vi "estimateKalmanRP.vi"(0 "Vision in":refnum<class "Vision.lvclass">, 1 "Robot ID":u32, 3 "Camera_id":enum16{"3", "2", "1", "0"}(ring), 4 "Click To continue":bool, 6 "Field Size":T2, 7 "Number of\nmeasurements\nper point":i32=1000, 9 "Team":enum16{"Azul", "Amarelo"}(ring) caption="Enum", 10 "NewCameras":T5[](array[typedef]) {"robots_blue"."height" format="%+4.3f"; "robots_blue"."pixel_y" format="%+4.3f"; "robots_blue"."pixel_x" format="%+4.3f"; "robots_blue"."orientation" format="%+4.3f"; "robots_blue"."y" format="%+4.3f"; "robots_blue"."confidence" format="%4.3f"; "robots_blue"."x" format="%+4.3f"; "robots_yellow"."height" format="%+4.3f"; "robots_yellow"."pixel_y" format="%+4.3f"; "robots_yellow"."pixel_x" format="%+4.3f"; "robots_yellow"."orientation" format="%+4.3f"; "robots_yellow"."y" format="%+4.3f"; "robots_yellow"."confidence" format="%4.3f"; "robots_yellow"."x" format="%+4.3f"}, 16 "ID Cameras Array":dbl[](array[numeric])) -> (11 "Current State":T3=enum."Canto inferior direito", 13 "Next State":T3=enum."Canto inferior direito", 14 "Vision out":refnum<class "Vision.lvclass">, 15 "Point Finished?":bool, 17 "Camera Finished?":bool, 18 "covariance matrix R":T4, 19 "covariance matrix P":T4)   [LabVIEW 2018, in "Vision.lvclass"]
uses:
  Vision.lvclass
  Old vision/Controls/SSL Detection Frame.ctl
  Old vision/Controls/SSL Detection Robot.ctl
  <vilib>/Analysis/Matrix/Datatypes/RealMatrix.ctl
  Old vision/Controls/SSL Detection Ball.ctl
  EstimateState.ctl
  EstimateLocation.ctl
  <vilib>/gmath/NI_Gmath.lvlib
  <vilib>/Analysis/Matrix/NI_Matrix.lvlib
panel:
  in  "Local":T1
  out "error out":errorcluster
  in  "error in (no error)":errorcluster
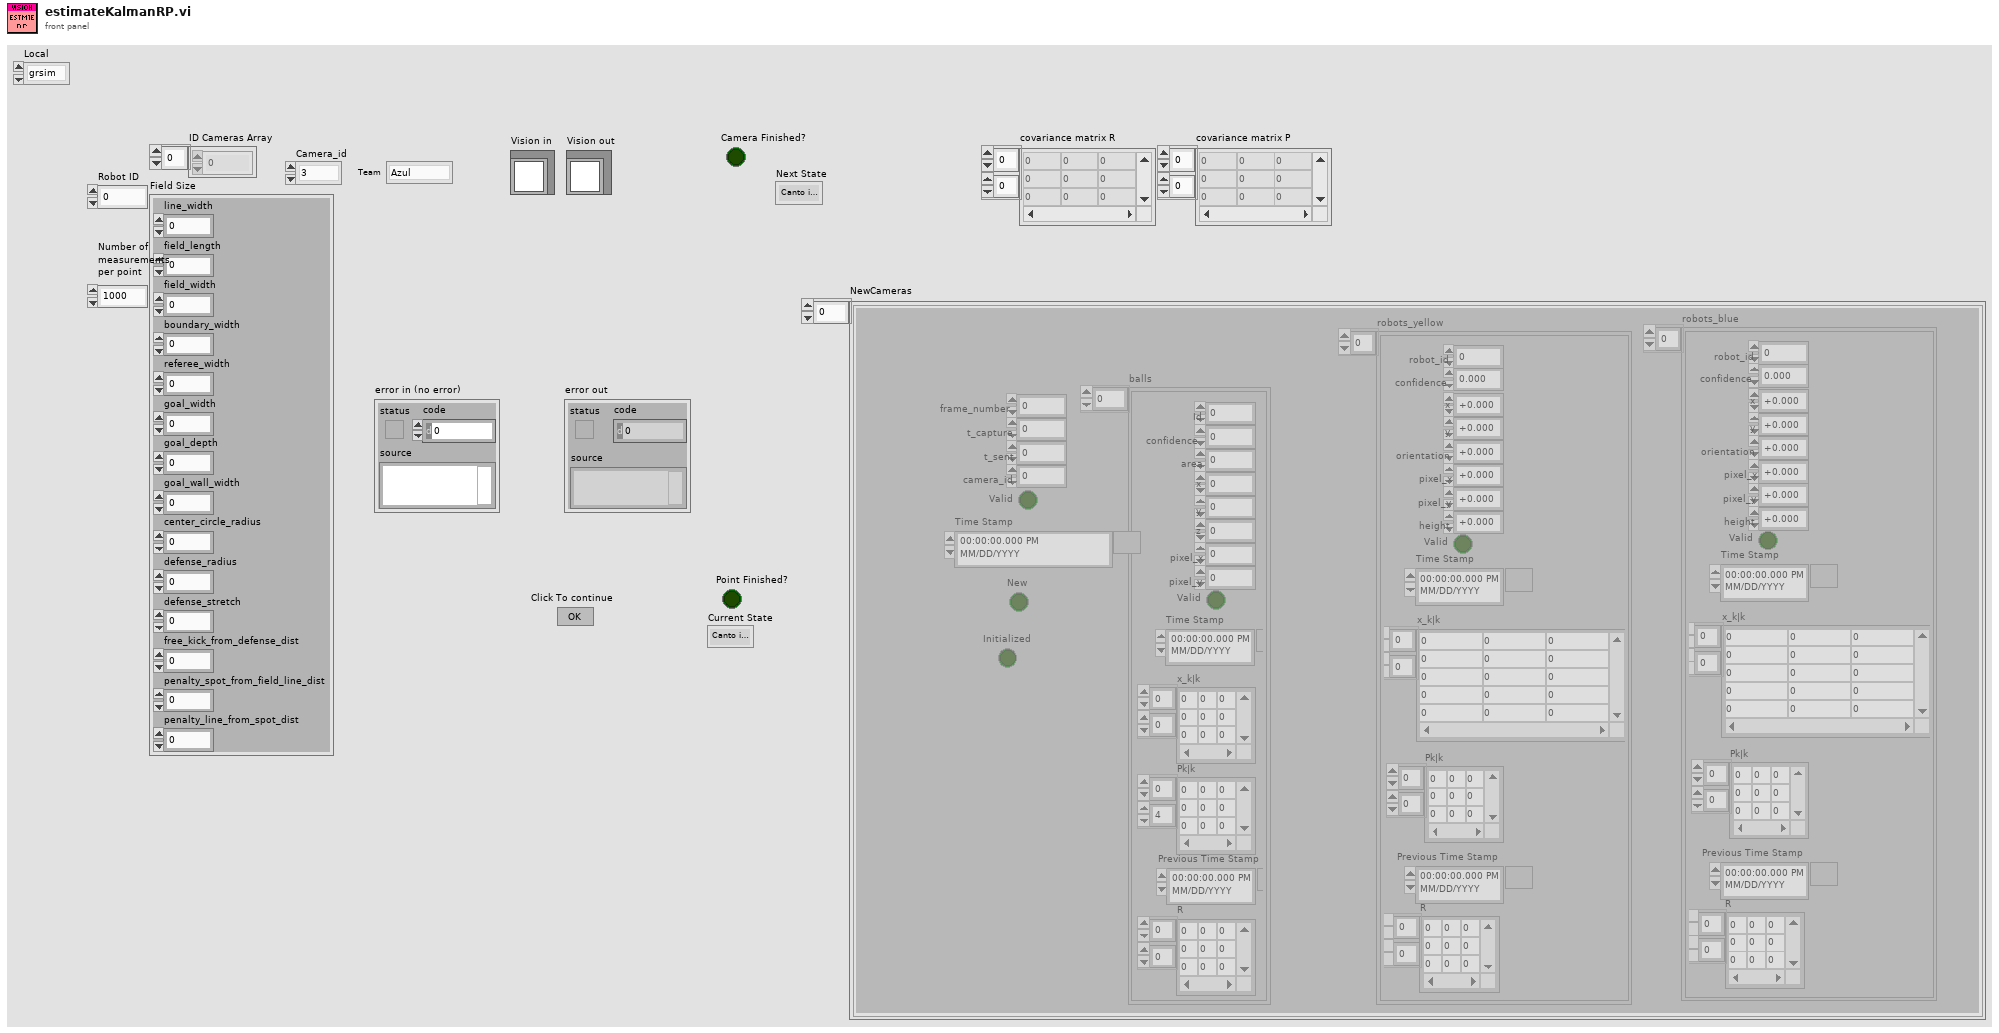
[diagram p1: front panel]
types:
  T1 = typedef "EstimateLocation.ctl" = enum16{"grsim", "RoboCup", "LARC"}
  T2 = cluster{"line_width":u32, "field_length":u32, "field_width":u32, "boundary_width":u32, "referee_width":u32, "goal_width":u32, "goal_depth":u32, "goal_wall_width":u32, "center_circle_radius":u32, "defense_radius":u32, "defense_stretch":u32, "free_kick_from_defense_dist":u32, "penalty_spot_from_field_line_dist":u32, "penalty_line_from_spot_dist":u32}
  T3 = typedef "EstimateState.ctl" = enum16{"Terminado", "Calculando", "Aguardando início", "Aguardando próximo passo", "Canto inferior direito", "Centro do gol direito", "Canto superior direito", "Meio superior", "Canto superior esquerdo", "Meio inferior", "Meio do campo", "Centro do gol esquerdo", "Canto inferior esquerdo", "Abaixo da câmera"}
  T4 = typedef "NI_Matrix.lvlib/RealMatrix.ctl" = dbl[][]
  T5 = typedef "SSL Detection Frame.ctl" = cluster{"frame_number":u32, "t_capture":dbl, "t_sent":dbl, "camera_id":u32, "robots_yellow":T6[], "robots_blue":T6[], "balls":T7[], "Valid":bool, "Time Stamp":timestamp, "New":bool, "Initialized":bool}
  T6 = typedef "SSL Detection Robot.ctl" = cluster{"x":sgl, "robot_id":u32, "confidence":sgl, "y":sgl, "orientation":sgl, "pixel_x":sgl, "pixel_y":sgl, "height":sgl, "Valid":bool, "Time Stamp":timestamp, "x_k|k":T4, "Pk|k":T4, "Previous Time Stamp":timestamp, "R":T4}
  T7 = typedef "SSL Detection Ball.ctl" = cluster{"x":sgl, "area":u32, "confidence":sgl, "y":sgl, "z":sgl, "pixel_x":sgl, "pixel_y":sgl, "Valid":bool, "Time Stamp":timestamp, "x_k|k":T4, "Pk|k":T4, "Id":u32, "Previous Time Stamp":timestamp, "R":T4}
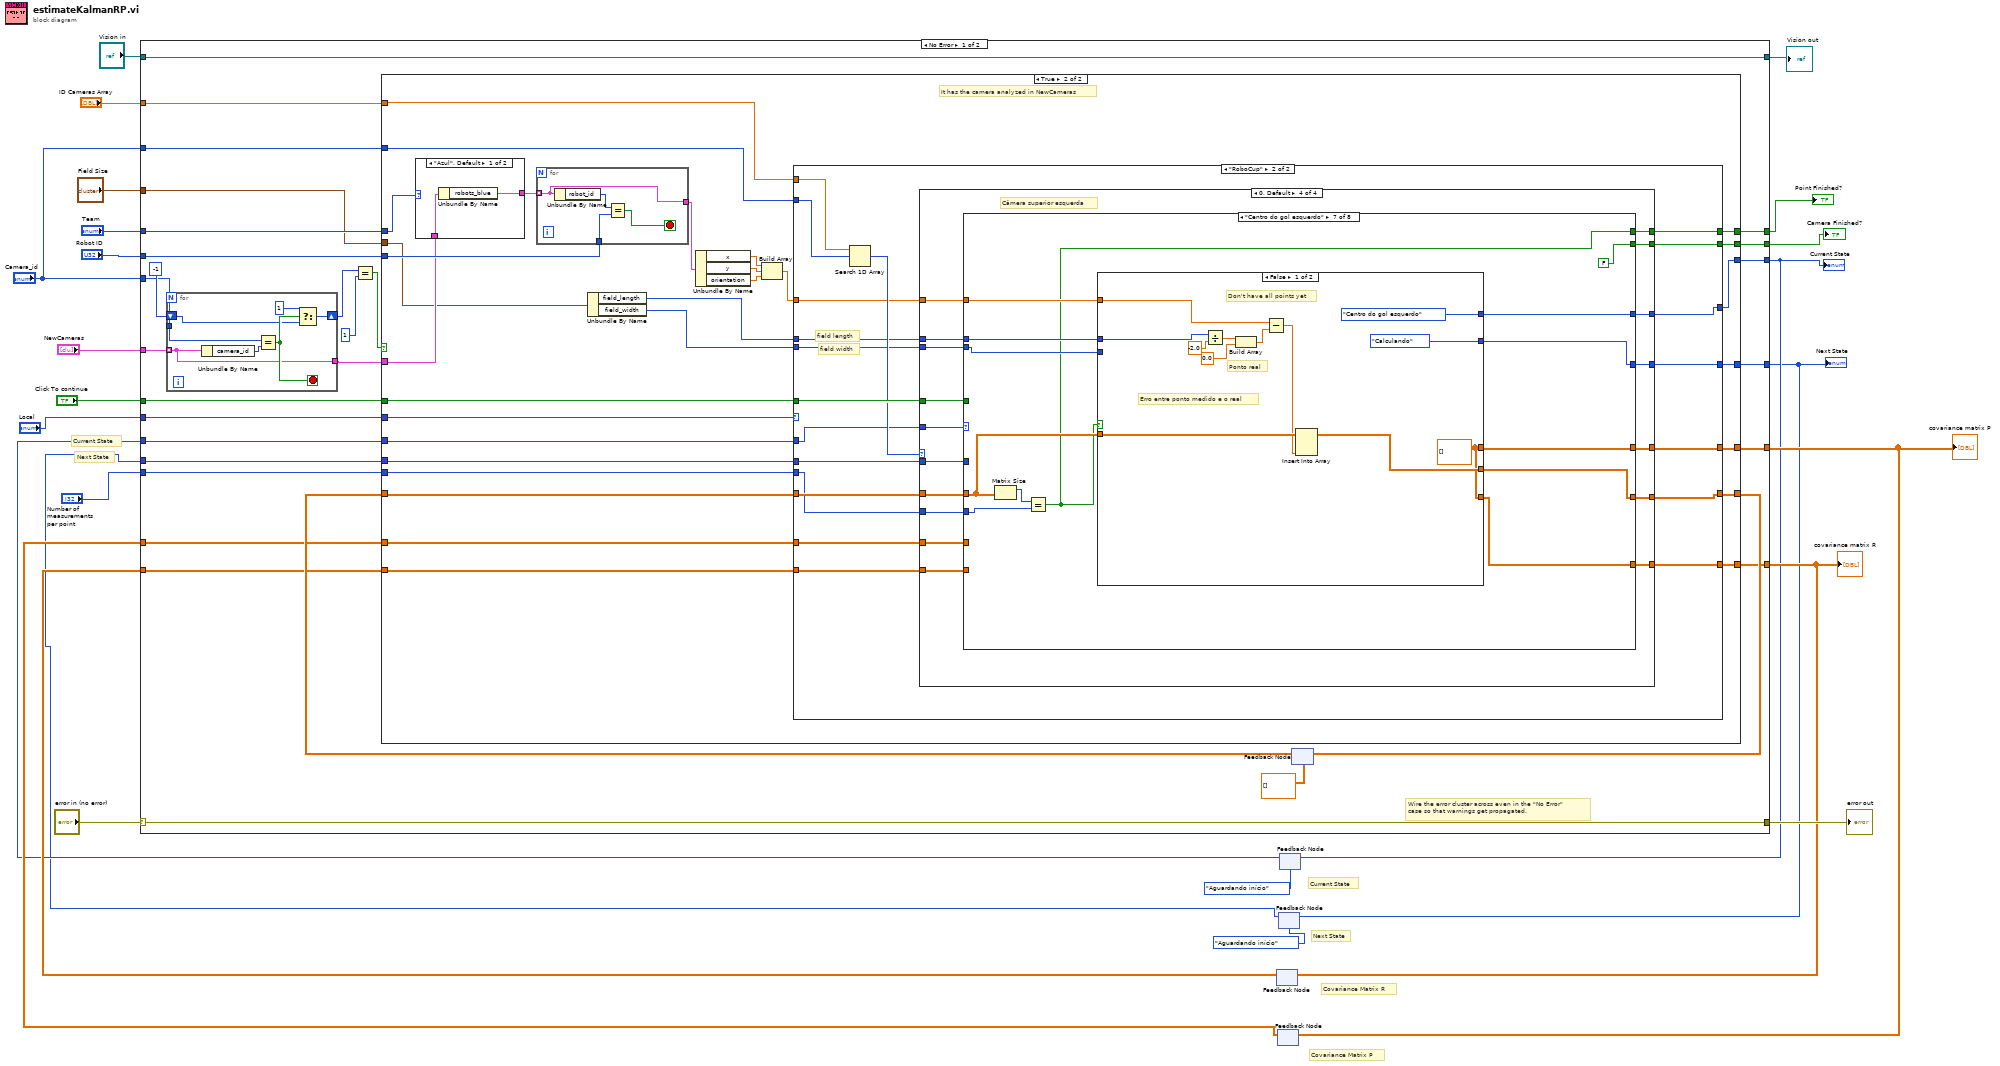
[diagram p0: block diagram]
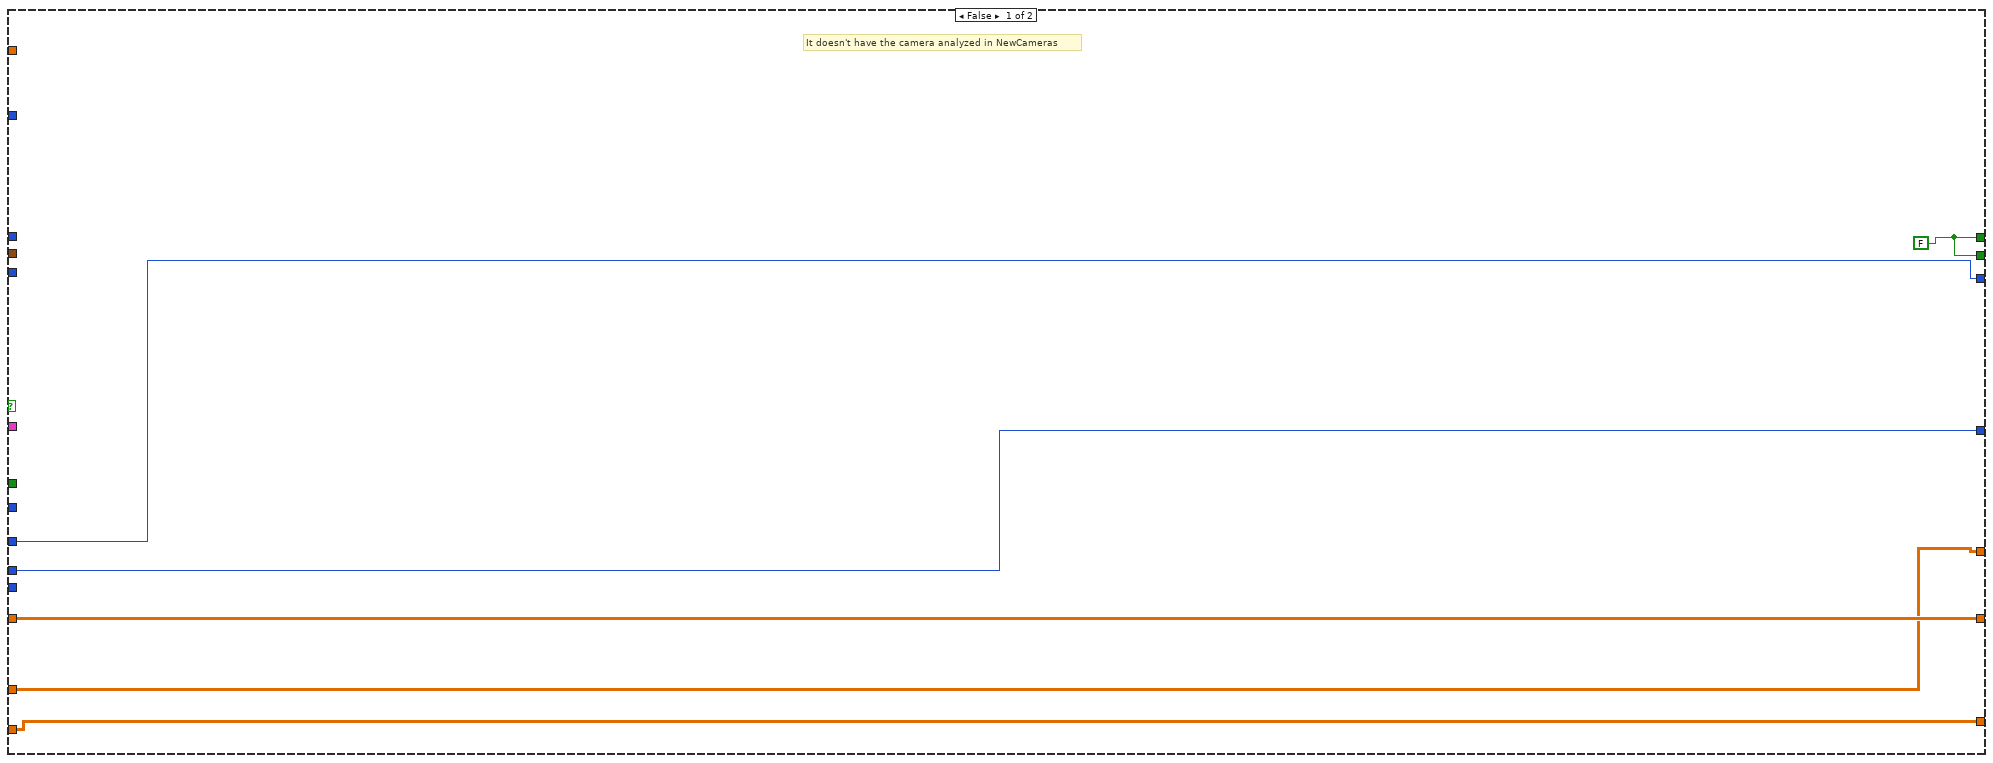
[diagram p2: hidden frame]
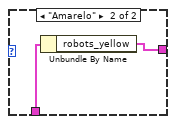
[diagram p3: hidden frame]
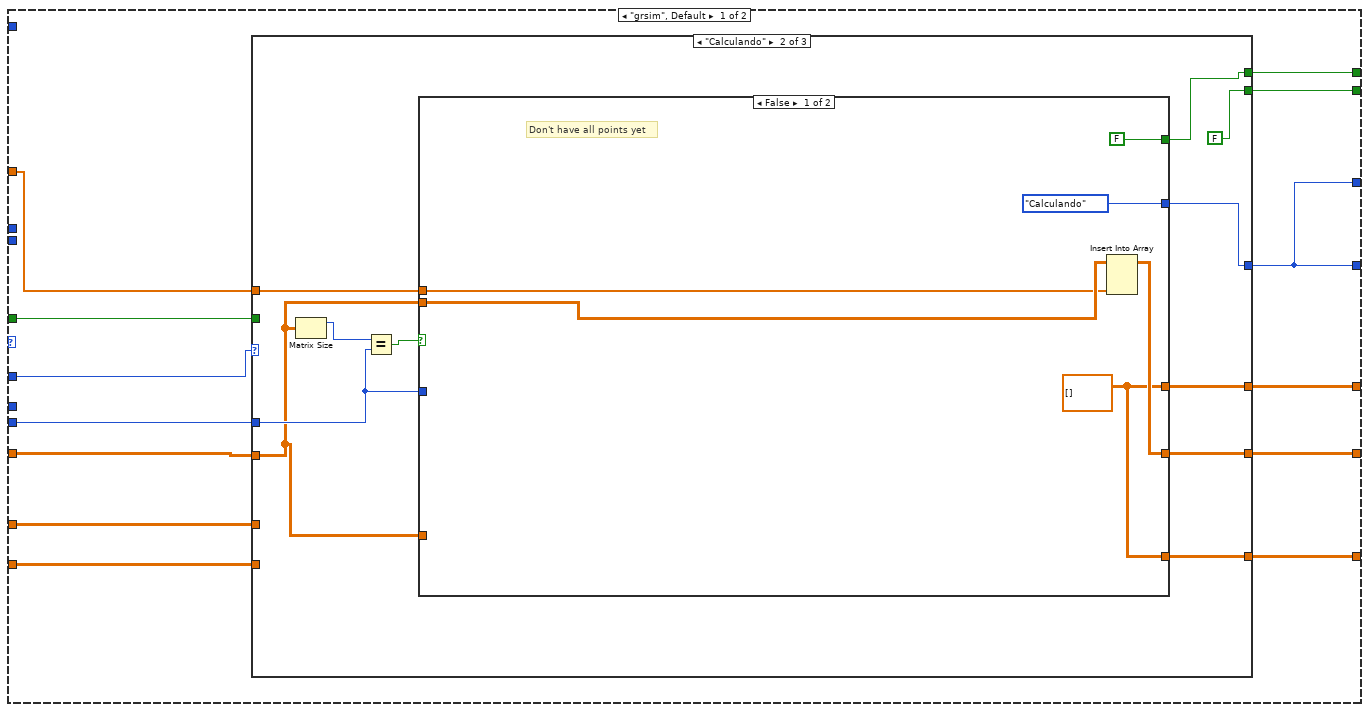
[diagram p4: hidden frame]
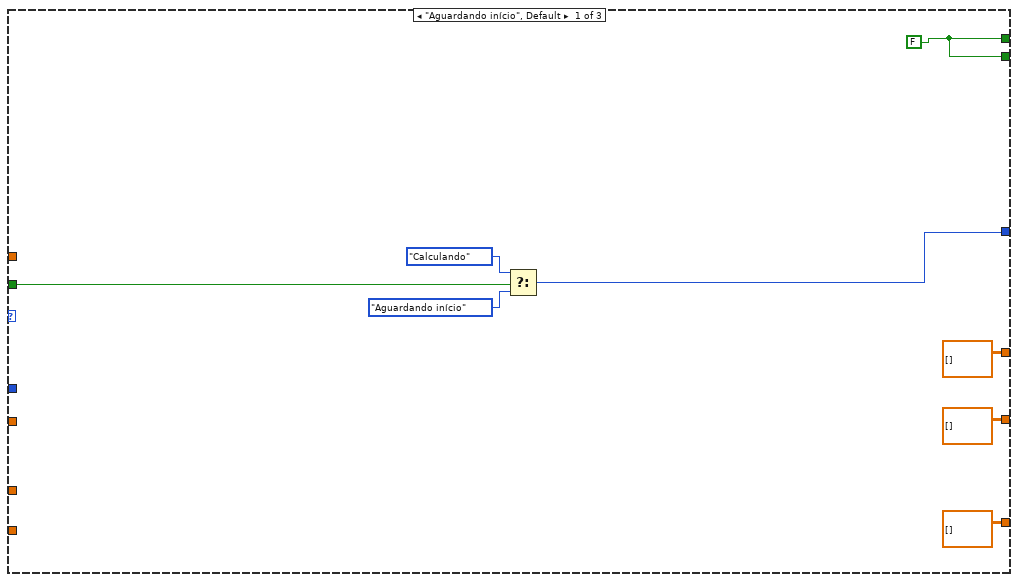
[diagram p5: hidden frame]
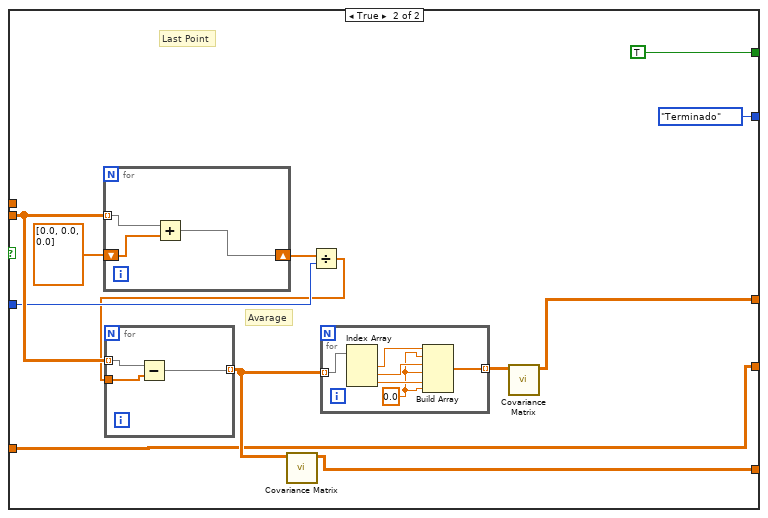
[diagram p6: hidden frame]
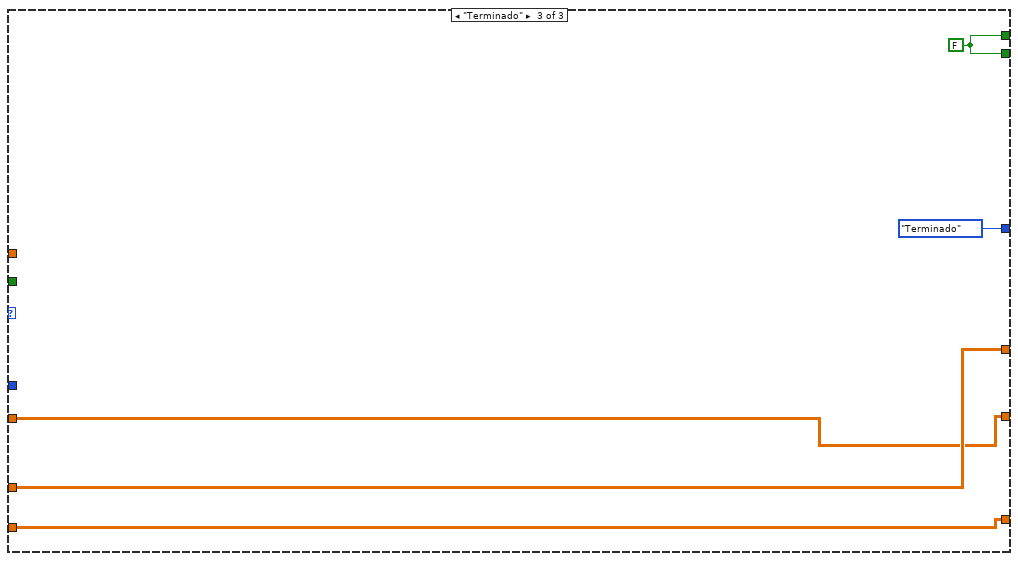
[diagram p7: hidden frame]
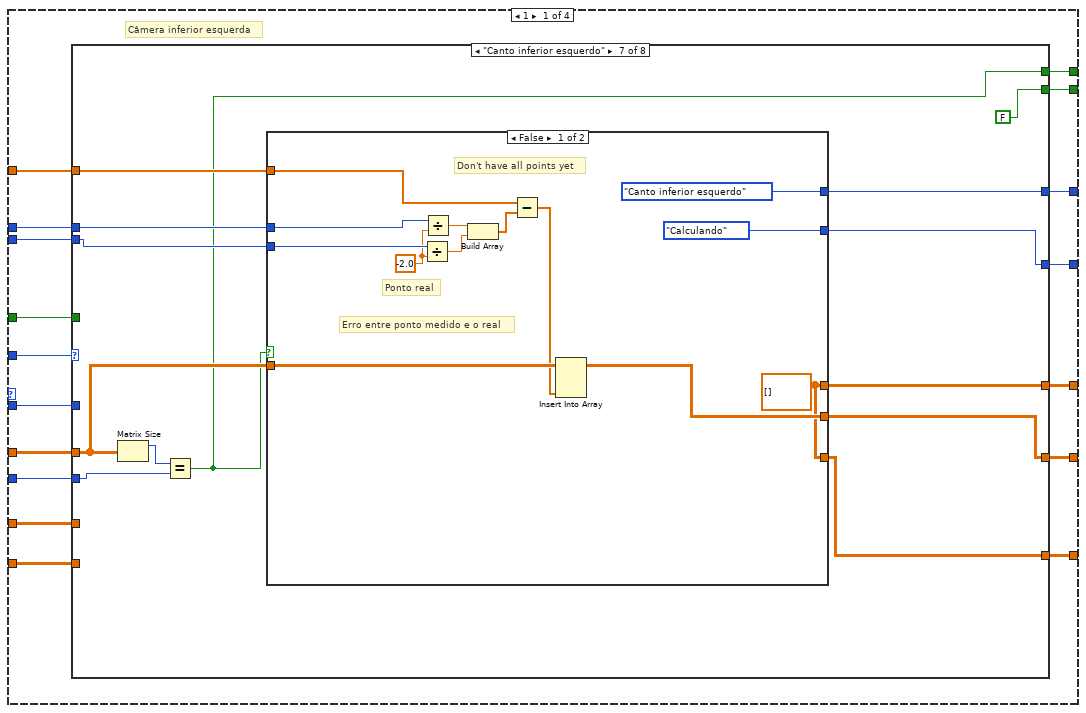
[diagram p8: hidden frame]
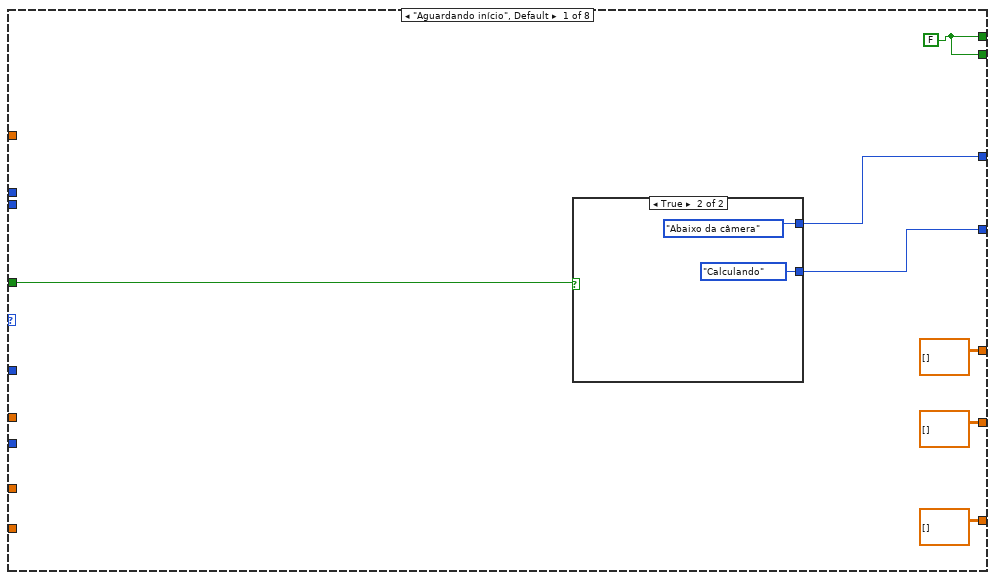
[diagram p9: hidden frame]
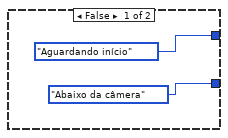
[diagram p10: hidden frame]
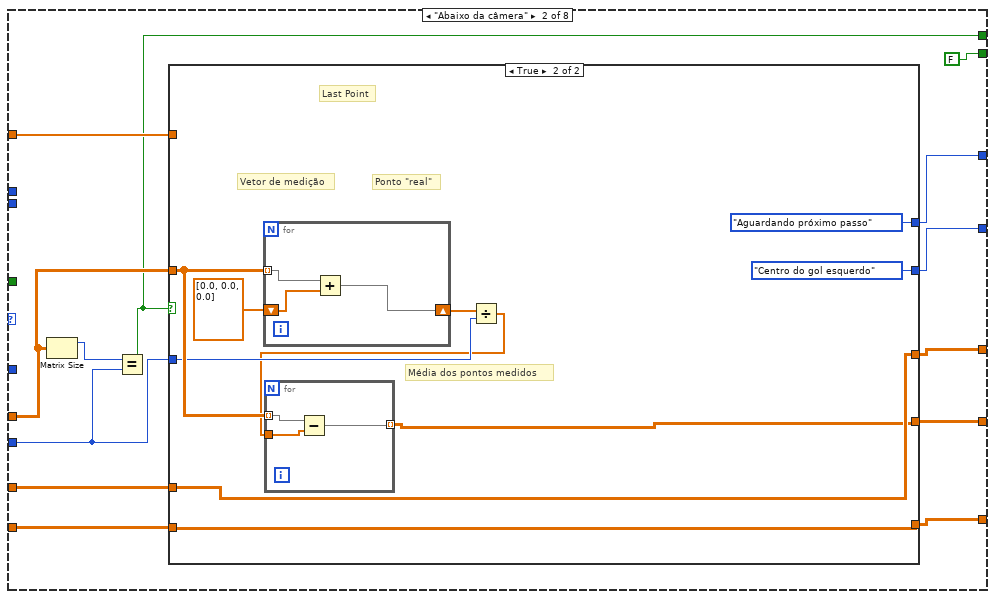
[diagram p11: hidden frame]
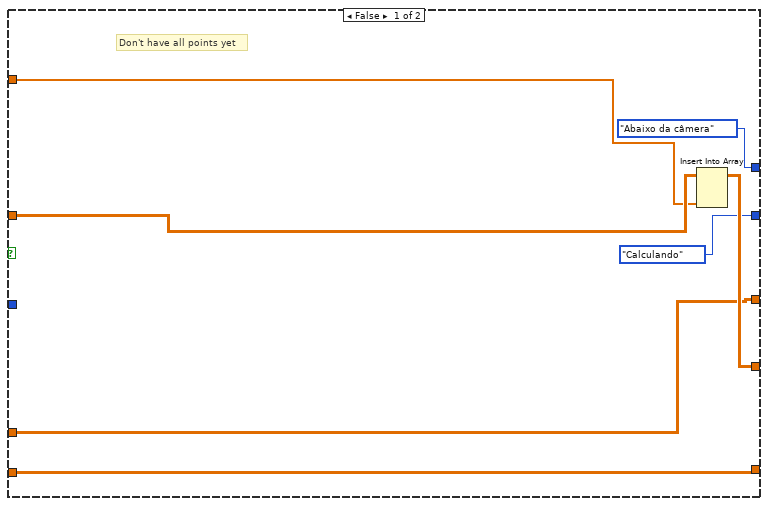
[diagram p12: hidden frame]
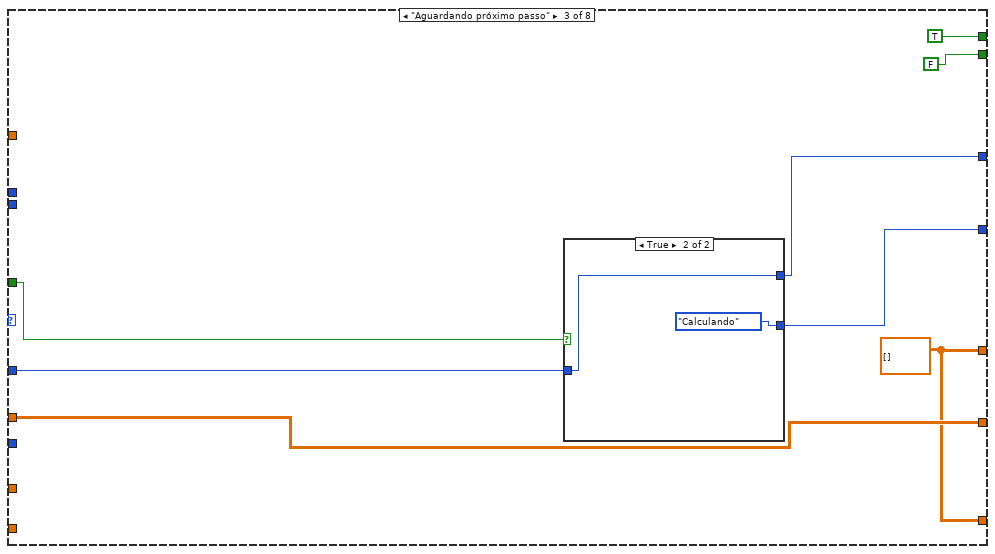
[diagram p13: hidden frame]
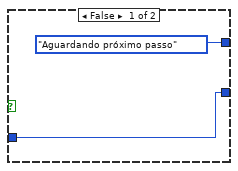
[diagram p14: hidden frame]
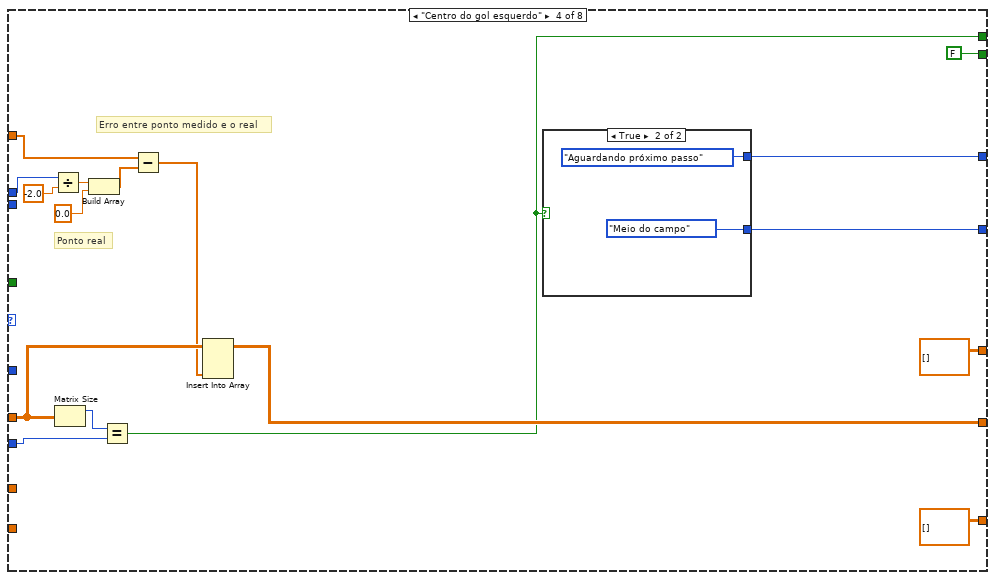
[diagram p15: hidden frame]
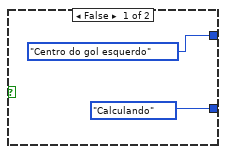
[diagram p16: hidden frame]
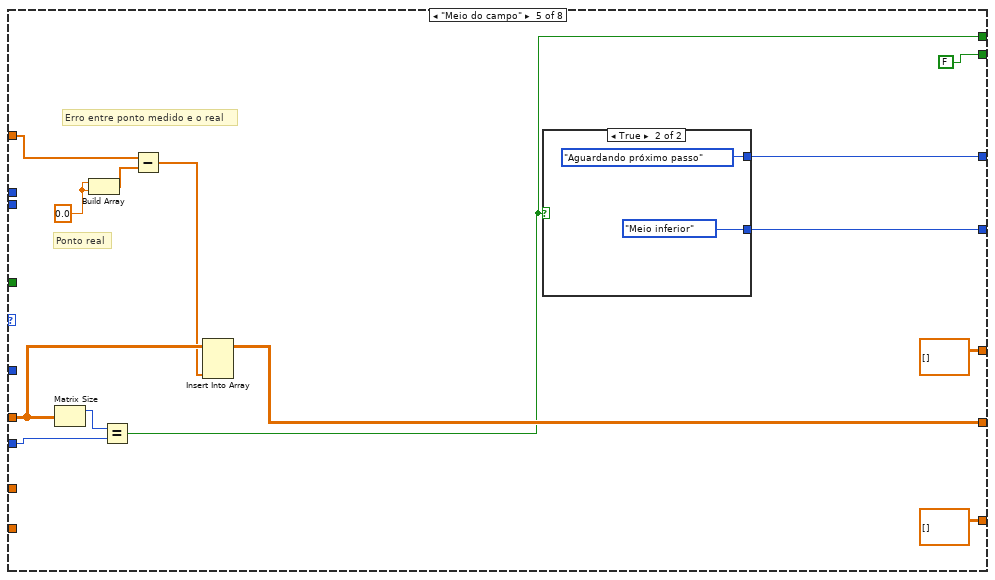
[diagram p17: hidden frame]
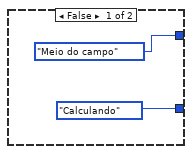
[diagram p18: hidden frame]
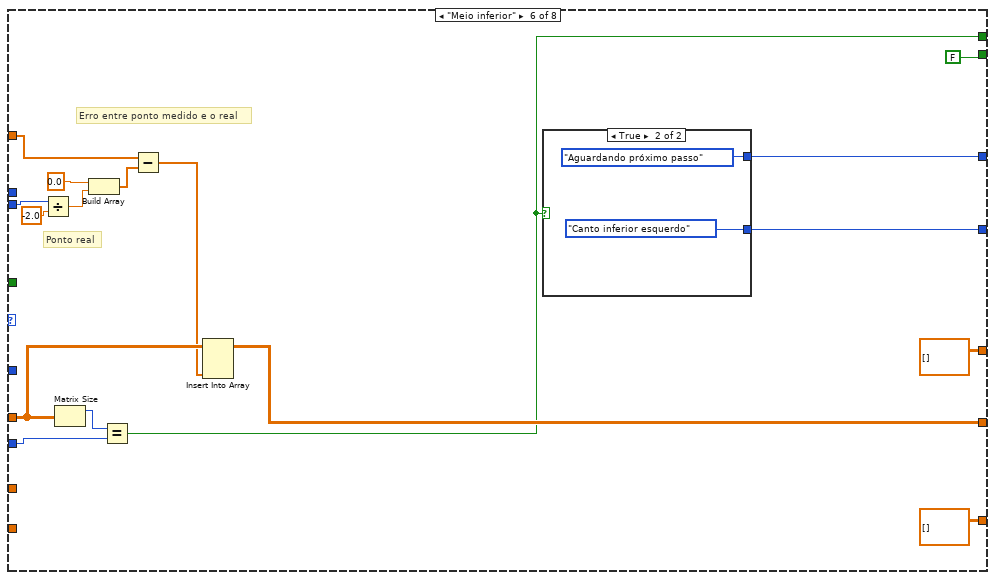
[diagram p19: hidden frame]
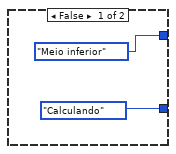
[diagram p20: hidden frame]
diagram:
  # "Next State"
  # "Current State"
  # "Next State"
  # "Current State"
  # "Covariance Matrix P"
  # "Covariance Matrix R"
  n1 = feedback #1() -> (w15:T4)  [unwired: 1 in]
  n2 = feedback #2() -> (w13:T4)  [unwired: 1 in]
  n3 = feedback #3(EstimateState."Aguardando início" ("State 2")) -> (w6:T3)
  n4 = feedback #4(EstimateState."Aguardando início" ("State 2")) -> (w9:T3)
  n5 = case shown="No Error" "error in (no error)" {
    selector: "error in (no error)" -> [w54 w909]
    tunnel: [w54 w909] -> w24
    tunnel: [w55 w908] -> w22
    tunnel: "Vision in" -> [w55 w908]
    tunnel: "Click To continue" -> [w53 _]
    tunnel: "Local" -> [w52 _]
    tunnel: "NewCameras" -> [w49 _]
    tunnel: "Number of\nmeasurements\nper point" -> [w51 _]
    tunnel: "Team" -> [w50 _]
    tunnel: "Camera_id" -> [w36 _]
    tunnel: [w40 _] -> w14
    tunnel: [w39 _] -> w16
    tunnel: w15 -> [w38 _]
    tunnel: w13 -> [w37 _]
    tunnel: "ID Cameras Array" -> [w35 _]
    tunnel: "Camera_id" -> [w34 _]
    tunnel: w9 -> [w33 _]
    tunnel: [w32 _] -> w8
    tunnel: [w31 _] -> w7
    tunnel: w6 -> [w30 _]
    tunnel: "Robot ID" -> [w29 _]
    tunnel: "Field Size" -> [w28 _]
    tunnel: [w27 _] -> w3
    tunnel: [w26 _] -> w2
    frame No Error {
      # "Wire the error cluster across even in the \"No Error\"\ncase so that warnings get propagated."
      n6 = for {
        tunnel: w49 -> [w901] mode=indexing
        tunnel: w36 -> [w906]
        shift-right: [w904] -> w47
        shift-left: -1 -> [w902]
        tunnel: [w901] -> w41
        stop <- w905 stop-if-true
        n7 = Unbundle By Name(w901) -> ("camera_id"=w907:u32)
        n8 = Equal?(x=w906, y=w907) -> (x = y?=w905:bool)
        n9 = Select(t=1, s=w905, f=w902) -> (s? t:f=w904:i32)
      }
      n10 = Equal?(x=w47, y=1) -> (x = y?=w46:bool)
      n11 = feedback #5(sgl[][] [] ("appended array")) -> (w42:dbl[][])
      n12 = case shown="True" w46 {
        tunnel: w53 -> [_ w90]
        tunnel: w52 -> [_ w89]
        tunnel: w51 -> [_ w88]
        tunnel: w50 -> [_ w74]
        tunnel: [w61 w86] -> w43
        tunnel: w42 -> [w61 w87]
        tunnel: w41 -> [_ w67]
        tunnel: [w60 w85] -> w40
        tunnel: [w59 w84] -> w39
        tunnel: w38 -> [w59 w83]
        tunnel: w37 -> [w60 w82]
        tunnel: w35 -> [_ w81]
        tunnel: w34 -> [_ w80]
        tunnel: w33 -> [w57 w79]
        tunnel: [w57 w78] -> w32
        tunnel: [w56 w77] -> w31
        tunnel: w30 -> [w56 w76]
        tunnel: w29 -> [_ w73]
        tunnel: w28 -> [_ w66]
        tunnel: [w58 w63] -> w27
        tunnel: [w58 w62] -> w26
        frame False {
          w58 = FALSE
          # "It doesn't have the camera analyzed in NewCameras"
        }
        frame True {
          # "It has the camera analyzed in NewCameras"
          n13 = case shown="\"Azul\", Default" w74 {
            tunnel: [w96 w98] -> w75
            tunnel: w67 -> [w95 w97]
            frame "Azul", Default {
              n14 = Unbundle By Name(w95) -> ("robots_blue"=w96:T6[])
            }
            frame "Amarelo" {
              n15 = Unbundle By Name(w97) -> ("robots_yellow"=w98:T6[])
            }
          }
          n16 = for {
            tunnel: w75 -> [w91] mode=indexing
            tunnel: w73 -> [w92]
            tunnel: [w91] -> w72
            stop <- w94 stop-if-true
            n17 = Unbundle By Name(w91) -> ("robot_id"=w93:u32)
            n18 = Equal?(x=w93, y=w92) -> (x = y?=w94:bool)
          }
          n19 = Unbundle By Name(w66) -> ("field_length"=w65:u32, "field_width"=w64:u32)
          n20 = Unbundle By Name(w72) -> ("x"=w71:sgl, "y"=w70:sgl, "orientation"=w69:sgl)
          n21 = Build Array(w71, w70, w69) -> (w68:sgl[])
          n22 = case shown="\"RoboCup\"" w89 {
            tunnel: w90 -> [w111 w185]
            tunnel: w88 -> [w110 w180]
            tunnel: w87 -> [w109 w181]
            tunnel: [w108 w179] -> w86
            tunnel: [w107 w178] -> w85
            tunnel: [w106 w177] -> w84
            tunnel: w83 -> [w105 w176]
            tunnel: w82 -> [w104 w175]
            tunnel: w81 -> [_ w184]
            tunnel: w80 -> [_ w183]
            tunnel: w79 -> [w103 w174]
            tunnel: [w102 w173] -> w78
            tunnel: [w102 w172] -> w77
            tunnel: w76 -> [_ w171]
            tunnel: w68 -> [w101 w170]
            tunnel: w65 -> [_ w169]
            tunnel: w64 -> [_ w168]
            tunnel: [w100 w167] -> w63
            tunnel: [w99 w166] -> w62
            frame "grsim", Default {
              n23 = case shown="\"Calculando\"" w103 {
                tunnel: w111 -> [w119 _ _]
                tunnel: [w116 w127 EstimateState."Terminado" ("State 2")] -> w102
                tunnel: w109 -> [_ w122 w162]
                tunnel: w110 -> [_ w126 _]
                tunnel: [dbl[][] [] ("appended array") w128 w162] -> w108
                tunnel: [T4 [] ("covariance matrix V") w125 w163] -> w107
                tunnel: [T4 [] ("covariance matrix V") w124 w165] -> w106
                tunnel: w105 -> [_ _ w165]
                tunnel: w104 -> [_ _ w163]
                tunnel: w101 -> [_ w123 _]
                tunnel: [w112 w121 w161] -> w100
                tunnel: [w112 FALSE w161] -> w99
                frame "Aguardando início", Default {
                  w112 = FALSE
                  n24 = Select(t=EstimateState."Calculando" ("State 2"), s=w119, f=EstimateState."Aguardando início" ("State 2")) -> (s? t:f=w116:T3)
                }
                frame "Calculando" {
                  n25 = Matrix Size(0:w122) -> (1:w130:i32)  [unwired: 1 out]
                  n26 = Equal?(x=w130, y=w126) -> (x = y?=w129:bool)
                  n27 = case shown="False" w129 {
                    tunnel: w122 -> [w136 w146]
                    tunnel: [w135 w138] -> w128
                    tunnel: [EstimateState."Calculando" ("State 2") EstimateState."Terminado" ("State 2")] -> w127
                    tunnel: w126 -> [_ w144]
                    tunnel: [w131 w140] -> w125
                    tunnel: [w131 w139] -> w124
                    tunnel: w123 -> [w133 _]
                    tunnel: w122 -> [_ w138]
                    tunnel: [FALSE TRUE] -> w121
                    frame False {
                      w131 = T4 [] ("covariance matrix V")
                      # "Don't have all points yet"
                      n28 = Insert Into Array(array=w136, new element=w133) -> (w135:dbl[][])  [unwired: 2 in]
                    }
                    frame True {
                      # "Avarage"
                      # "Last Point"
                      n29 = for {
                        tunnel: w146 -> [w160] mode=indexing
                        shift-right: [w159] -> w145
                        shift-left: sgl[] [0.0, 0.0, 0.0] ("appended array") -> [w158]
                        n30 = Add(x=w160, y=w158) -> (x+y=w159:dbl[])
                      }
                      n31 = Divide(x=w145, y=w144) -> (x/y=w143:dbl[])
                      n32 = for {
                        tunnel: w146 -> [w157] mode=indexing
                        tunnel: w143 -> [w156]
                        tunnel: [w155] -> w142 mode=indexing
                        n33 = Subtract(x=w157, y=w156) -> (x-y=w155:dbl[])
                      }
                      n34 = call <vilib>:"Covariance Matrix.vi"("X"=w142) -> ("covariance matrix V"=w139:T4)  [unwired: 9 in, 1 out]
                      n35 = for {
                        tunnel: w142 -> [w154] mode=indexing
                        tunnel: [w149] -> w141 mode=indexing
                        w150 = 0.0
                        n36 = Index Array(array=w154) -> (element #1=w153:dbl, element #2=w152:dbl, element #3=w151:dbl)  [unwired: 3 in]
                        n37 = Build Array(w153, w150, w152, w150, w151, w150) -> (w149:dbl[])
                      }
                      n38 = call <vilib>:"Covariance Matrix.vi"("X"=w141) -> ("covariance matrix V"=w140:T4)  [unwired: 9 in, 1 out]
                    }
                  }
                }
                frame "Terminado" {
                  w161 = FALSE
                }
              }
            }
            frame "RoboCup" {
              # "field width"
              # "field length"
              n39 = Search 1D Array(1D array=w184, element=w183) -> (index of element=w182:i32)  [unwired: 1 in]
              n40 = case shown="0, Default" w182 {
                tunnel: w185 -> [w202 w380 w559 w738]
                tunnel: w181 -> [w201 w379 w558 w737]
                tunnel: w180 -> [w200 w378 w557 w736]
                tunnel: [w199 w377 w556 w735] -> w179
                tunnel: [w198 w376 w555 w734] -> w178
                tunnel: [w197 w375 w554 w733] -> w177
                tunnel: w176 -> [w196 w374 w553 w732]
                tunnel: w175 -> [w195 w373 w552 w731]
                tunnel: w174 -> [w194 w372 w551 w730]
                tunnel: [w193 w371 w550 w729] -> w173
                tunnel: [w192 w370 w549 w728] -> w172
                tunnel: w171 -> [w191 w369 w548 w727]
                tunnel: w170 -> [w190 w368 w547 w726]
                tunnel: w169 -> [w189 w367 w546 w725]
                tunnel: w168 -> [w188 w366 w545 w724]
                tunnel: [w187 w365 w544 w723] -> w167
                tunnel: [w186 w364 w543 w722] -> w166
                frame 1 {
                  # "Câmera inferior esquerda"
                  n41 = case shown="\"Canto inferior esquerdo\"" w194 {
                    tunnel: w202 -> [w209 _ w257 _ _ _ _ _]
                    tunnel: w201 -> [_ w225 w253 w270 w292 w314 w331 w363]
                    tunnel: w200 -> [_ w224 _ w277 w295 w316 w333 _]
                    tunnel: [dbl[][] [] ("appended array") w223 w253 w268 w290 w312 w326 w363] -> w199
                    tunnel: [T4 [] ("covariance matrix V") w222 w252 T4 [] ("covariance matrix V") T4 [] ("covariance matrix V") T4 [] ("covariance matrix V") w328 w362] -> w198
                    tunnel: [T4 [] ("covariance matrix V") w221 w252 T4 [] ("covariance matrix V") T4 [] ("covariance matrix V") T4 [] ("covariance matrix V") w327 w361] -> w197
                    tunnel: w196 -> [_ w220 _ _ _ _ _ w361]
                    tunnel: w195 -> [_ w219 _ _ _ _ _ w362]
                    tunnel: [w208 w218 w256 w264 w286 w308 w324 w360] -> w193
                    tunnel: [w207 w217 w254 w265 w287 w309 w325 w360] -> w192
                    tunnel: w191 -> [_ _ w255 _ _ _ _ _]
                    tunnel: w190 -> [_ w216 _ w276 w294 w315 w332 _]
                    tunnel: w189 -> [_ _ _ w274 _ _ w329 _]
                    tunnel: w188 -> [_ _ _ _ _ w303 w330 _]
                    tunnel: [w203 w215 TRUE w263 w284 w302 w323 w359] -> w187
                    tunnel: [w203 FALSE FALSE FALSE FALSE FALSE FALSE w359] -> w186
                    frame "Aguardando início", Default {
                      w203 = FALSE
                      n42 = case shown="True" w209 {
                        tunnel: [EstimateState."Aguardando início" ("State 2") EstimateState."Abaixo da câmera" ("State 2")] -> w208
                        tunnel: [EstimateState."Abaixo da câmera" ("State 2") EstimateState."Calculando" ("State 2")] -> w207
                        frame False {
                        }
                        frame True {
                        }
                      }
                    }
                    frame "Abaixo da câmera" {
                      n43 = Matrix Size(0:w225) -> (1:w226:i32)  [unwired: 1 out]
                      n44 = Equal?(x=w226, y=w224) -> (x = y?=w215:bool)
                      n45 = case shown="True" w215 {
                        tunnel: w225 -> [w233 w242]
                        tunnel: [w232 w234] -> w223
                        tunnel: w224 -> [_ w240]
                        tunnel: [w230 w235] -> w222
                        tunnel: [w231 w236] -> w221
                        tunnel: w220 -> [w231 w236]
                        tunnel: w219 -> [w230 w235]
                        tunnel: [EstimateState."Calculando" ("State 2") EstimateState."Centro do gol esquerdo" ("State 2")] -> w217
                        tunnel: [EstimateState."Abaixo da câmera" ("State 2") EstimateState."Aguardando próximo passo" ("State 2")] -> w218
                        tunnel: w216 -> [w227 _]
                        frame False {
                          # "Don't have all points yet"
                          n46 = Insert Into Array(array=w233, new element=w227) -> (w232:dbl[][])  [unwired: 2 in]
                        }
                        frame True {
                          # "Ponto \"real\""
                          # "Vetor de medição"
                          # "Média dos pontos medidos"
                          # "Last Point"
                          n47 = for {
                            tunnel: w242 -> [w249] mode=indexing
                            shift-right: [w248] -> w241
                            shift-left: sgl[] [0.0, 0.0, 0.0] ("appended array") -> [w247]
                            n48 = Add(x=w249, y=w247) -> (x+y=w248:dbl[])
                          }
                          n49 = Divide(x=w241, y=w240) -> (x/y=w239:dbl[])
                          n50 = for {
                            tunnel: w242 -> [w246] mode=indexing
                            tunnel: w239 -> [w245]
                            tunnel: [w244] -> w234 mode=indexing
                            n51 = Subtract(x=w246, y=w245) -> (x-y=w244:dbl[])
                          }
                        }
                      }
                    }
                    frame "Aguardando próximo passo" {
                      w252 = T4 [] ("covariance matrix V")
                      n52 = case shown="True" w257 {
                        tunnel: [EstimateState."Aguardando próximo passo" ("Current State 2") w260] -> w256
                        tunnel: [w258 EstimateState."Calculando" ("Current State 2")] -> w254
                        tunnel: w255 -> [w258 w260]
                        frame False {
                        }
                        frame True {
                        }
                      }
                    }
                    frame "Centro do gol esquerdo" {
                      # "Erro entre ponto medido e o real"
                      # "Ponto real"
                      n53 = Divide(x=w274, y=-2.0) -> (x/y=w272:dbl)
                      n54 = Matrix Size(0:w270) -> (1:w278:i32)  [unwired: 1 out]
                      n55 = Build Array(w272, 0.0) -> (w275:dbl[])
                      n56 = Equal?(x=w278, y=w277) -> (x = y?=w263:bool)
                      n57 = Subtract(x=w276, y=w275) -> (x-y=w269:dbl[])
                      n58 = Insert Into Array(array=w270, new element=w269) -> (w268:dbl[][])  [unwired: 2 in]
                      n59 = case shown="True" w263 {
                        tunnel: [EstimateState."Calculando" ("Current State 2") EstimateState."Meio do campo" ("Current State 2")] -> w265
                        tunnel: [EstimateState."Centro do gol esquerdo" ("Current State 2") EstimateState."Aguardando próximo passo" ("Current State 2")] -> w264
                        frame False {
                        }
                        frame True {
                        }
                      }
                    }
                    frame "Meio do campo" {
                      w285 = 0.0
                      # "Ponto real"
                      # "Erro entre ponto medido e o real"
                      n60 = Matrix Size(0:w292) -> (1:w296:i32)  [unwired: 1 out]
                      n61 = Build Array(w285, w285) -> (w293:dbl[])
                      n62 = Equal?(x=w296, y=w295) -> (x = y?=w284:bool)
                      n63 = Subtract(x=w294, y=w293) -> (x-y=w291:dbl[])
                      n64 = Insert Into Array(array=w292, new element=w291) -> (w290:dbl[][])  [unwired: 2 in]
                      n65 = case shown="True" w284 {
                        tunnel: [EstimateState."Calculando" ("Current State 2") EstimateState."Meio inferior" ("Current State 2")] -> w287
                        tunnel: [EstimateState."Meio do campo" ("Current State 2") EstimateState."Aguardando próximo passo" ("Current State 2")] -> w286
                        frame False {
                        }
                        frame True {
                        }
                      }
                    }
                    frame "Meio inferior" {
                      # "Ponto real"
                      # "Erro entre ponto medido e o real"
                      n66 = Divide(x=w303, y=-2.0) -> (x/y=w305:dbl)
                      n67 = Matrix Size(0:w314) -> (1:w317:i32)  [unwired: 1 out]
                      n68 = Build Array(0.0, w305) -> (w306:dbl[])
                      n69 = Equal?(x=w317, y=w316) -> (x = y?=w302:bool)
                      n70 = Subtract(x=w315, y=w306) -> (x-y=w313:dbl[])
                      n71 = Insert Into Array(array=w314, new element=w313) -> (w312:dbl[][])  [unwired: 2 in]
                      n72 = case shown="True" w302 {
                        tunnel: [EstimateState."Calculando" ("Current State 2") EstimateState."Canto inferior esquerdo" ("Current State 2")] -> w309
                        tunnel: [EstimateState."Meio inferior" ("Current State 2") EstimateState."Aguardando próximo passo" ("Current State 2")] -> w308
                        frame False {
                        }
                        frame True {
                        }
                      }
                    }
                    frame "Canto inferior esquerdo" {
                      n73 = Matrix Size(0:w331) -> (1:w334:i32)  [unwired: 1 out]
                      n74 = Equal?(x=w334, y=w333) -> (x = y?=w323:bool)
                      n75 = case shown="False" w323 {
                        tunnel: w332 -> [w347 _]
                        tunnel: w331 -> [w346 w349]
                        tunnel: [w337 w350] -> w327
                        tunnel: w330 -> [w342 _]
                        tunnel: w329 -> [w341 _]
                        tunnel: [w337 w351] -> w328
                        tunnel: [w338 w349] -> w326
                        tunnel: [EstimateState."Calculando" ("Current State 2") w348] -> w325
                        tunnel: [EstimateState."Canto inferior esquerdo" ("Current State 2") w348] -> w324
                        frame False {
                          w337 = T4 [] ("covariance matrix V")
                          w340 = -2.0 ("y")
                          # "Ponto real"
                          # "Erro entre ponto medido e o real"
                          # "Don't have all points yet"
                          n76 = Divide(x=w342, y=w340) -> (x/y=w343:dbl)
                          n77 = Divide(x=w341, y=w340) -> (x/y=w339:dbl)
                          n78 = Build Array(w339, w343) -> (w344:dbl[])
                          n79 = Subtract(x=w347, y=w344) -> (x-y=w345:dbl[])
                          n80 = Insert Into Array(array=w346, new element=w345) -> (w338:dbl[][])  [unwired: 2 in]
                        }
                        frame True {
                          w348 = EstimateState."Terminado" ("Current State 2")
                          # "Estimate R"
                          # "Estimate P"
                          # "Last Point"
                          n81 = for {
                            tunnel: w349 -> [w358] mode=indexing
                            tunnel: [w353] -> w352 mode=indexing
                            w354 = 0.0
                            n82 = Index Array(array=w358) -> (element #1=w357:dbl, element #2=w356:dbl, element #3=w355:dbl)  [unwired: 3 in]
                            n83 = Build Array(w357, w354, w356, w354, w355, w354) -> (w353:dbl[])
                          }
                          n84 = call <vilib>:"Covariance Matrix.vi"("X"=w349) -> ("covariance matrix V"=w350:T4)  [unwired: 9 in, 1 out]
                          n85 = call <vilib>:"Covariance Matrix.vi"("X"=w352) -> ("covariance matrix V"=w351:T4)  [unwired: 9 in, 1 out]
                        }
                      }
                    }
                    frame "Terminado" {
                      w359 = TRUE
                      w360 = EstimateState."Terminado" ("Current State 2")
                    }
                  }
                }
                frame 2 {
                  # "Câmera inferior direita"
                  n86 = case shown="\"Meio inferior\"" w372 {
                    tunnel: w380 -> [w387 _ w435 _ _ _ _ _]
                    tunnel: w379 -> [_ w403 w431 w449 w470 w494 w511 w542]
                    tunnel: w378 -> [_ w402 _ w452 w473 w496 w513 _]
                    tunnel: [dbl[][] [] ("appended array") w401 w431 w447 w468 w492 w506 w542] -> w377
                    tunnel: [T4 [] ("covariance matrix V") w400 w430 T4 [] ("covariance matrix V") T4 [] ("covariance matrix V") T4 [] ("covariance matrix V") w508 w541] -> w376
                    tunnel: [T4 [] ("covariance matrix V") w399 w430 T4 [] ("covariance matrix V") T4 [] ("covariance matrix V") T4 [] ("covariance matrix V") w507 w540] -> w375
                    tunnel: w374 -> [_ w398 _ _ _ _ _ w540]
                    tunnel: w373 -> [_ w397 _ _ _ _ _ w541]
                    tunnel: [w386 w396 w434 w443 w464 w488 w504 w539] -> w371
                    tunnel: [w385 w395 w432 w444 w465 w489 w505 w539] -> w370
                    tunnel: w369 -> [_ _ w433 _ _ _ _ _]
                    tunnel: w368 -> [_ w394 _ w451 w472 w495 w512 _]
                    tunnel: w367 -> [_ _ _ _ w460 w481 w509 _]
                    tunnel: w366 -> [_ _ _ _ _ w484 w510 _]
                    tunnel: [w381 w393 TRUE w442 w462 w483 w503 w538] -> w365
                    tunnel: [w381 FALSE FALSE FALSE FALSE FALSE FALSE w538] -> w364
                    frame "Aguardando início", Default {
                      w381 = FALSE
                      n87 = case shown="True" w387 {
                        tunnel: [EstimateState."Aguardando início" ("State 2") EstimateState."Abaixo da câmera" ("State 2")] -> w386
                        tunnel: [EstimateState."Abaixo da câmera" ("State 2") EstimateState."Calculando" ("State 2")] -> w385
                        frame False {
                        }
                        frame True {
                        }
                      }
                    }
                    frame "Abaixo da câmera" {
                      n88 = Matrix Size(0:w403) -> (1:w404:i32)  [unwired: 1 out]
                      n89 = Equal?(x=w404, y=w402) -> (x = y?=w393:bool)
                      n90 = case shown="True" w393 {
                        tunnel: w403 -> [w411 w420]
                        tunnel: [w410 w412] -> w401
                        tunnel: w402 -> [_ w418]
                        tunnel: [w408 w413] -> w400
                        tunnel: [w409 w414] -> w399
                        tunnel: w398 -> [w409 w414]
                        tunnel: w397 -> [w408 w413]
                        tunnel: [EstimateState."Calculando" ("State 2") EstimateState."Meio do campo" ("State 2")] -> w395
                        tunnel: [EstimateState."Abaixo da câmera" ("State 2") EstimateState."Aguardando próximo passo" ("State 2")] -> w396
                        tunnel: w394 -> [w405 _]
                        frame False {
                          # "Don't have all points yet"
                          n91 = Insert Into Array(array=w411, new element=w405) -> (w410:dbl[][])  [unwired: 2 in]
                        }
                        frame True {
                          # "Ponto \"real\""
                          # "Vetor de medição"
                          # "Média dos pontos medidos"
                          # "Last Point"
                          n92 = for {
                            tunnel: w420 -> [w427] mode=indexing
                            shift-right: [w426] -> w419
                            shift-left: sgl[] [0.0, 0.0, 0.0] ("appended array") -> [w425]
                            n93 = Add(x=w427, y=w425) -> (x+y=w426:dbl[])
                          }
                          n94 = Divide(x=w419, y=w418) -> (x/y=w417:dbl[])
                          n95 = for {
                            tunnel: w420 -> [w424] mode=indexing
                            tunnel: w417 -> [w423]
                            tunnel: [w422] -> w412 mode=indexing
                            n96 = Subtract(x=w424, y=w423) -> (x-y=w422:dbl[])
                          }
                        }
                      }
                    }
                    frame "Aguardando próximo passo" {
                      w430 = T4 [] ("covariance matrix V")
                      n97 = case shown="True" w435 {
                        tunnel: [EstimateState."Aguardando próximo passo" ("Current State 2") w438] -> w434
                        tunnel: [w436 EstimateState."Calculando" ("Current State 2")] -> w432
                        tunnel: w433 -> [w436 w438]
                        frame False {
                        }
                        frame True {
                        }
                      }
                    }
                    frame "Meio do campo" {
                      w440 = 0.0
                      # "Erro entre ponto medido e o real"
                      # "Ponto real"
                      n98 = Matrix Size(0:w449) -> (1:w453:i32)  [unwired: 1 out]
                      n99 = Build Array(w440, w440) -> (w450:dbl[])
                      n100 = Equal?(x=w453, y=w452) -> (x = y?=w442:bool)
                      n101 = Subtract(x=w451, y=w450) -> (x-y=w448:dbl[])
                      n102 = Insert Into Array(array=w449, new element=w448) -> (w447:dbl[][])  [unwired: 2 in]
                      n103 = case shown="True" w442 {
                        tunnel: [EstimateState."Calculando" ("Current State 2") EstimateState."Centro do gol direito" ("Current State 2")] -> w444
                        tunnel: [EstimateState."Meio do campo" ("Current State 2") EstimateState."Aguardando próximo passo" ("Current State 2")] -> w443
                        frame False {
                        }
                        frame True {
                        }
                      }
                    }
                    frame "Centro do gol direito" {
                      # "Ponto real"
                      # "Erro entre ponto medido e o real"
                      n104 = Divide(x=w460, y=2.0) -> (x/y=w458:dbl)
                      n105 = Matrix Size(0:w470) -> (1:w474:i32)  [unwired: 1 out]
                      n106 = Build Array(w458, 0.0) -> (w471:dbl[])
                      n107 = Equal?(x=w474, y=w473) -> (x = y?=w462:bool)
                      n108 = Subtract(x=w472, y=w471) -> (x-y=w469:dbl[])
                      n109 = Insert Into Array(array=w470, new element=w469) -> (w468:dbl[][])  [unwired: 2 in]
                      n110 = case shown="True" w462 {
                        tunnel: [EstimateState."Calculando" ("Current State 2") EstimateState."Canto inferior direito" ("Current State 2")] -> w465
                        tunnel: [EstimateState."Centro do gol direito" ("Current State 2") EstimateState."Aguardando próximo passo" ("Current State 2")] -> w464
                        frame False {
                        }
                        frame True {
                        }
                      }
                    }
                    frame "Canto inferior direito" {
                      # "Ponto real"
                      # "Erro entre ponto medido e o real"
                      n111 = Divide(x=w484, y=-2.0) -> (x/y=w486:dbl)
                      n112 = Divide(x=w481, y=2.0) -> (x/y=w479:dbl)
                      n113 = Matrix Size(0:w494) -> (1:w497:i32)  [unwired: 1 out]
                      n114 = Build Array(w479, w486) -> (w487:dbl[])
                      n115 = Equal?(x=w497, y=w496) -> (x = y?=w483:bool)
                      n116 = Subtract(x=w495, y=w487) -> (x-y=w493:dbl[])
                      n117 = Insert Into Array(array=w494, new element=w493) -> (w492:dbl[][])  [unwired: 2 in]
                      n118 = case shown="True" w483 {
                        tunnel: [EstimateState."Calculando" ("Current State 2") EstimateState."Meio inferior" ("Current State 2")] -> w489
                        tunnel: [EstimateState."Canto inferior direito" ("Current State 2") EstimateState."Aguardando próximo passo" ("Current State 2")] -> w488
                        frame False {
                        }
                        frame True {
                        }
                      }
                    }
                    frame "Meio inferior" {
                      n119 = Matrix Size(0:w511) -> (1:w514:i32)  [unwired: 1 out]
                      n120 = Equal?(x=w514, y=w513) -> (x = y?=w503:bool)
                      n121 = case shown="False" w503 {
                        tunnel: w512 -> [w526 _]
                        tunnel: w511 -> [w525 w528]
                        tunnel: [w518 w529] -> w507
                        tunnel: w510 -> [w521 _]
                        tunnel: w509 -> [_ _]
                        tunnel: [w518 w530] -> w508
                        tunnel: [w519 w528] -> w506
                        tunnel: [EstimateState."Calculando" ("Current State 2") w527] -> w505
                        tunnel: [EstimateState."Meio inferior" ("Current State 2") w527] -> w504
                        frame False {
                          w518 = T4 [] ("covariance matrix V")
                          # "Ponto real"
                          # "Erro entre ponto medido e o real"
                          # "Don't have all points yet"
                          n122 = Divide(x=w521, y=-2.0) -> (x/y=w522:dbl)
                          n123 = Build Array(0.0 ("y"), w522) -> (w523:dbl[])
                          n124 = Subtract(x=w526, y=w523) -> (x-y=w524:dbl[])
                          n125 = Insert Into Array(array=w525, new element=w524) -> (w519:dbl[][])  [unwired: 2 in]
                        }
                        frame True {
                          w527 = EstimateState."Terminado" ("Current State 2")
                          # "Estimate R"
                          # "Estimate P"
                          # "Last Point"
                          n126 = for {
                            tunnel: w528 -> [w537] mode=indexing
                            tunnel: [w532] -> w531 mode=indexing
                            w533 = 0.0
                            n127 = Index Array(array=w537) -> (element #1=w536:dbl, element #2=w535:dbl, element #3=w534:dbl)  [unwired: 3 in]
                            n128 = Build Array(w536, w533, w535, w533, w534, w533) -> (w532:dbl[])
                          }
                          n129 = call <vilib>:"Covariance Matrix.vi"("X"=w528) -> ("covariance matrix V"=w529:T4)  [unwired: 9 in, 1 out]
                          n130 = call <vilib>:"Covariance Matrix.vi"("X"=w531) -> ("covariance matrix V"=w530:T4)  [unwired: 9 in, 1 out]
                        }
                      }
                    }
                    frame "Terminado" {
                      w538 = TRUE
                      w539 = EstimateState."Terminado" ("Current State 2")
                    }
                  }
                }
                frame 3 {
                  # "Câmera superior direita"
                  n131 = case shown="\"Aguardando início\", Default" w551 {
                    tunnel: w559 -> [w566 _ w614 _ _ _ _ _]
                    tunnel: w558 -> [_ w582 w610 w631 w654 w676 w693 w721]
                    tunnel: w557 -> [_ w581 _ w634 w657 w678 w695 _]
                    tunnel: [dbl[][] [] ("appended array") w580 w610 w629 w652 w674 w688 w721] -> w556
                    tunnel: [T4 [] ("covariance matrix V") w579 w609 T4 [] ("covariance matrix V") T4 [] ("covariance matrix V") T4 [] ("covariance matrix V") w690 w720] -> w555
                    tunnel: [T4 [] ("covariance matrix V") w578 w609 T4 [] ("covariance matrix V") T4 [] ("covariance matrix V") T4 [] ("covariance matrix V") w689 w719] -> w554
                    tunnel: w553 -> [_ w577 _ _ _ _ _ w719]
                    tunnel: w552 -> [_ w576 _ _ _ _ _ w720]
                    tunnel: [w565 w575 w613 w625 w648 w670 w686 w718] -> w550
                    tunnel: [w564 w574 w611 w626 w649 w671 w687 w718] -> w549
                    tunnel: w548 -> [_ _ w612 _ _ _ _ _]
                    tunnel: w547 -> [_ w573 _ w633 w656 w677 w694 _]
                    tunnel: w546 -> [_ _ _ w621 w645 w666 w691 _]
                    tunnel: w545 -> [_ _ _ _ w642 _ w692 _]
                    tunnel: [w560 w572 TRUE w624 w647 w668 w685 w717] -> w544
                    tunnel: [w560 FALSE FALSE FALSE FALSE FALSE FALSE w717] -> w543
                    frame "Aguardando início", Default {
                      w560 = FALSE
                      n132 = case shown="False" w566 {
                        tunnel: [EstimateState."Aguardando início" ("State 2") EstimateState."Abaixo da câmera" ("State 2")] -> w565
                        tunnel: [EstimateState."Abaixo da câmera" ("State 2") EstimateState."Calculando" ("State 2")] -> w564
                        frame False {
                        }
                        frame True {
                        }
                      }
                    }
                    frame "Abaixo da câmera" {
                      n133 = Matrix Size(0:w582) -> (1:w583:i32)  [unwired: 1 out]
                      n134 = Equal?(x=w583, y=w581) -> (x = y?=w572:bool)
                      n135 = case shown="True" w572 {
                        tunnel: w582 -> [w590 w599]
                        tunnel: [w589 w591] -> w580
                        tunnel: w581 -> [_ w597]
                        tunnel: [w587 w592] -> w579
                        tunnel: [w588 w593] -> w578
                        tunnel: w577 -> [w588 w593]
                        tunnel: w576 -> [w587 w592]
                        tunnel: [EstimateState."Calculando" ("State 2") EstimateState."Meio superior" ("State 2")] -> w574
                        tunnel: [EstimateState."Abaixo da câmera" ("State 2") EstimateState."Aguardando próximo passo" ("State 2")] -> w575
                        tunnel: w573 -> [w584 _]
                        frame False {
                          # "Don't have all points yet"
                          n136 = Insert Into Array(array=w590, new element=w584) -> (w589:dbl[][])  [unwired: 2 in]
                        }
                        frame True {
                          # "Ponto \"real\""
                          # "Vetor de medição"
                          # "Média dos pontos medidos"
                          # "Last Point"
                          n137 = for {
                            tunnel: w599 -> [w606] mode=indexing
                            shift-right: [w605] -> w598
                            shift-left: sgl[] [0.0, 0.0, 0.0] ("appended array") -> [w604]
                            n138 = Add(x=w606, y=w604) -> (x+y=w605:dbl[])
                          }
                          n139 = Divide(x=w598, y=w597) -> (x/y=w596:dbl[])
                          n140 = for {
                            tunnel: w599 -> [w603] mode=indexing
                            tunnel: w596 -> [w602]
                            tunnel: [w601] -> w591 mode=indexing
                            n141 = Subtract(x=w603, y=w602) -> (x-y=w601:dbl[])
                          }
                        }
                      }
                    }
                    frame "Aguardando próximo passo" {
                      w609 = T4 [] ("covariance matrix V")
                      n142 = case shown="True" w614 {
                        tunnel: [EstimateState."Aguardando próximo passo" ("Current State 2") w617] -> w613
                        tunnel: [w615 EstimateState."Calculando" ("Current State 2")] -> w611
                        tunnel: w612 -> [w615 w617]
                        frame False {
                        }
                        frame True {
                        }
                      }
                    }
                    frame "Meio superior" {
                      # "Erro entre ponto medido e o real"
                      # "Ponto real"
                      n143 = Divide(x=w621, y=2.0) -> (x/y=w619:dbl)
                      n144 = Matrix Size(0:w631) -> (1:w635:i32)  [unwired: 1 out]
                      n145 = Build Array(w619, 0.0) -> (w632:dbl[])
                      n146 = Equal?(x=w635, y=w634) -> (x = y?=w624:bool)
                      n147 = Subtract(x=w633, y=w632) -> (x-y=w630:dbl[])
                      n148 = Insert Into Array(array=w631, new element=w630) -> (w629:dbl[][])  [unwired: 2 in]
                      n149 = case shown="True" w624 {
                        tunnel: [EstimateState."Calculando" ("Current State 2") EstimateState."Canto superior direito" ("Current State 2")] -> w626
                        tunnel: [EstimateState."Meio superior" ("Current State 2") EstimateState."Aguardando próximo passo" ("Current State 2")] -> w625
                        frame False {
                        }
                        frame True {
                        }
                      }
                    }
                    frame "Canto superior direito" {
                      # "Ponto real"
                      # "Erro entre ponto medido e o real"
                      n150 = Divide(x=w645, y=2.0) -> (x/y=w643:dbl)
                      n151 = Divide(x=w642, y=2.0) -> (x/y=w640:dbl)
                      n152 = Matrix Size(0:w654) -> (1:w658:i32)  [unwired: 1 out]
                      n153 = Build Array(w643, w640) -> (w655:dbl[])
                      n154 = Equal?(x=w658, y=w657) -> (x = y?=w647:bool)
                      n155 = Subtract(x=w656, y=w655) -> (x-y=w653:dbl[])
                      n156 = Insert Into Array(array=w654, new element=w653) -> (w652:dbl[][])  [unwired: 2 in]
                      n157 = case shown="True" w647 {
                        tunnel: [EstimateState."Calculando" ("Current State 2") EstimateState."Centro do gol direito" ("Current State 2")] -> w649
                        tunnel: [EstimateState."Canto superior direito" ("Current State 2") EstimateState."Aguardando próximo passo" ("Current State 2")] -> w648
                        frame False {
                        }
                        frame True {
                        }
                      }
                    }
                    frame "Centro do gol direito" {
                      # "Ponto real"
                      # "Erro entre ponto medido e o real"
                      n158 = Divide(x=w666, y=2.0) -> (x/y=w664:dbl)
                      n159 = Matrix Size(0:w676) -> (1:w679:i32)  [unwired: 1 out]
                      n160 = Build Array(w664, 0.0 ("y")) -> (w669:dbl[])
                      n161 = Equal?(x=w679, y=w678) -> (x = y?=w668:bool)
                      n162 = Subtract(x=w677, y=w669) -> (x-y=w675:dbl[])
                      n163 = Insert Into Array(array=w676, new element=w675) -> (w674:dbl[][])  [unwired: 2 in]
                      n164 = case shown="True" w668 {
                        tunnel: [EstimateState."Calculando" ("Current State 2") EstimateState."Meio do campo" ("Current State 2")] -> w671
                        tunnel: [EstimateState."Centro do gol direito" ("Current State 2") EstimateState."Aguardando próximo passo" ("Current State 2")] -> w670
                        frame False {
                        }
                        frame True {
                        }
                      }
                    }
                    frame "Meio do campo" {
                      n165 = Matrix Size(0:w693) -> (1:w696:i32)  [unwired: 1 out]
                      n166 = Equal?(x=w696, y=w695) -> (x = y?=w685:bool)
                      n167 = case shown="False" w685 {
                        tunnel: w694 -> [w705 _]
                        tunnel: w693 -> [w704 w707]
                        tunnel: [w700 w708] -> w689
                        tunnel: w692 -> [_ _]
                        tunnel: w691 -> [_ _]
                        tunnel: [w700 w709] -> w690
                        tunnel: [w701 w707] -> w688
                        tunnel: [EstimateState."Calculando" ("Current State 2") w706] -> w687
                        tunnel: [EstimateState."Meio do campo" ("Current State 2") w706] -> w686
                        frame False {
                          w697 = 0.0 ("y")
                          w700 = T4 [] ("covariance matrix V")
                          # "Ponto real"
                          # "Erro entre ponto medido e o real"
                          # "Don't have all points yet"
                          n168 = Build Array(w697, w697) -> (w702:dbl[])
                          n169 = Subtract(x=w705, y=w702) -> (x-y=w703:dbl[])
                          n170 = Insert Into Array(array=w704, new element=w703) -> (w701:dbl[][])  [unwired: 2 in]
                        }
                        frame True {
                          w706 = EstimateState."Terminado" ("Current State 2")
                          # "Estimate R"
                          # "Estimate P"
                          # "Last Point"
                          n171 = for {
                            tunnel: w707 -> [w716] mode=indexing
                            tunnel: [w711] -> w710 mode=indexing
                            w712 = 0.0
                            n172 = Index Array(array=w716) -> (element #1=w715:dbl, element #2=w714:dbl, element #3=w713:dbl)  [unwired: 3 in]
                            n173 = Build Array(w715, w712, w714, w712, w713, w712) -> (w711:dbl[])
                          }
                          n174 = call <vilib>:"Covariance Matrix.vi"("X"=w707) -> ("covariance matrix V"=w708:T4)  [unwired: 9 in, 1 out]
                          n175 = call <vilib>:"Covariance Matrix.vi"("X"=w710) -> ("covariance matrix V"=w709:T4)  [unwired: 9 in, 1 out]
                        }
                      }
                    }
                    frame "Terminado" {
                      w717 = TRUE
                      w718 = EstimateState."Terminado" ("Current State 2")
                    }
                  }
                }
                frame 0, Default {
                  # "Câmera superior esquerda"
                  n176 = case shown="\"Centro do gol esquerdo\"" w730 {
                    tunnel: w738 -> [w745 _ w793 _ _ _ _ _]
                    tunnel: w737 -> [_ w761 w789 w809 w834 w852 w869 w900]
                    tunnel: w736 -> [_ w760 _ w815 w836 w854 w871 _]
                    tunnel: [dbl[][] [] ("appended array") w759 w789 w807 w832 w850 w864 w900] -> w735
                    tunnel: [T4 [] ("covariance matrix V") w758 w788 T4 [] ("covariance matrix V") T4 [] ("covariance matrix V") T4 [] ("covariance matrix V") w866 w899] -> w734
                    tunnel: [T4 [] ("covariance matrix V") w757 w788 T4 [] ("covariance matrix V") T4 [] ("covariance matrix V") T4 [] ("covariance matrix V") w865 w898] -> w733
                    tunnel: w732 -> [_ w756 _ _ _ _ _ w898]
                    tunnel: w731 -> [_ w755 _ _ _ _ _ w899]
                    tunnel: [w744 w754 w792 w803 w828 w846 w862 w897] -> w729
                    tunnel: [w743 w753 w790 w804 w829 w847 w863 w897] -> w728
                    tunnel: w727 -> [_ _ w791 _ _ _ _ _]
                    tunnel: w726 -> [_ w752 _ w814 w835 w853 w870 _]
                    tunnel: w725 -> [_ _ _ w812 _ _ w867 _]
                    tunnel: w724 -> [_ _ _ w800 w824 _ w868 _]
                    tunnel: [w739 w751 TRUE w802 w827 w844 w861 w896] -> w723
                    tunnel: [w739 FALSE FALSE FALSE FALSE FALSE FALSE w896] -> w722
                    frame "Aguardando início", Default {
                      w739 = FALSE
                      n177 = case shown="True" w745 {
                        tunnel: [EstimateState."Aguardando início" ("State 2") EstimateState."Abaixo da câmera" ("State 2")] -> w744
                        tunnel: [EstimateState."Abaixo da câmera" ("State 2") EstimateState."Calculando" ("State 2")] -> w743
                        frame False {
                        }
                        frame True {
                        }
                      }
                    }
                    frame "Abaixo da câmera" {
                      n178 = Matrix Size(0:w761) -> (1:w762:i32)  [unwired: 1 out]
                      n179 = Equal?(x=w762, y=w760) -> (x = y?=w751:bool)
                      n180 = case shown="True" w751 {
                        tunnel: w761 -> [w769 w778]
                        tunnel: [w768 w770] -> w759
                        tunnel: w760 -> [_ w776]
                        tunnel: [w766 w771] -> w758
                        tunnel: [w767 w772] -> w757
                        tunnel: w756 -> [w767 w772]
                        tunnel: w755 -> [w766 w771]
                        tunnel: [EstimateState."Calculando" ("State 2") EstimateState."Canto superior esquerdo" ("State 2")] -> w753
                        tunnel: [EstimateState."Abaixo da câmera" ("State 2") EstimateState."Aguardando próximo passo" ("State 2")] -> w754
                        tunnel: w752 -> [w763 _]
                        frame False {
                          # "Don't have all points yet"
                          n181 = Insert Into Array(array=w769, new element=w763) -> (w768:dbl[][])  [unwired: 2 in]
                        }
                        frame True {
                          # "Ponto \"real\""
                          # "Vetor de medidas"
                          # "Média dos pontos medidos"
                          # "Last Point"
                          n182 = for {
                            tunnel: w778 -> [w785] mode=indexing
                            shift-right: [w784] -> w777
                            shift-left: sgl[] [0.0, 0.0, 0.0] ("appended array") -> [w783]
                            n183 = Add(x=w785, y=w783) -> (x+y=w784:dbl[])
                          }
                          n184 = Divide(x=w777, y=w776) -> (x/y=w775:dbl[])
                          n185 = for {
                            tunnel: w778 -> [w782] mode=indexing
                            tunnel: w775 -> [w781]
                            tunnel: [w780] -> w770 mode=indexing
                            n186 = Subtract(x=w782, y=w781) -> (x-y=w780:dbl[])
                          }
                        }
                      }
                    }
                    frame "Aguardando próximo passo" {
                      w788 = T4 [] ("covariance matrix V")
                      n187 = case shown="True" w793 {
                        tunnel: [EstimateState."Aguardando próximo passo" ("Current State 2") w796] -> w792
                        tunnel: [w794 EstimateState."Calculando" ("Current State 2")] -> w790
                        tunnel: w791 -> [w794 w796]
                        frame False {
                        }
                        frame True {
                        }
                      }
                    }
                    frame "Canto superior esquerdo" {
                      # "Erro entre ponto medido e o real"
                      # "Ponto real"
                      n188 = Divide(x=w800, y=2.0) -> (x/y=w798:dbl)
                      n189 = Divide(x=w812, y=-2.0) -> (x/y=w810:dbl)
                      n190 = Matrix Size(0:w809) -> (1:w816:i32)  [unwired: 1 out]
                      n191 = Build Array(w810, w798) -> (w813:dbl[])
                      n192 = Equal?(x=w816, y=w815) -> (x = y?=w802:bool)
                      n193 = Subtract(x=w814, y=w813) -> (x-y=w808:dbl[])
                      n194 = Insert Into Array(array=w809, new element=w808) -> (w807:dbl[][])  [unwired: 2 in]
                      n195 = case shown="True" w802 {
                        tunnel: [EstimateState."Calculando" ("Current State 2") EstimateState."Meio superior" ("Current State 2")] -> w804
                        tunnel: [EstimateState."Canto superior esquerdo" ("Current State 2") EstimateState."Aguardando próximo passo" ("Current State 2")] -> w803
                        frame False {
                        }
                        frame True {
                        }
                      }
                    }
                    frame "Meio superior" {
                      # "Erro entre ponto medido e o real"
                      # "Ponto real"
                      n196 = Divide(x=w824, y=2.0) -> (x/y=w822:dbl)
                      n197 = Matrix Size(0:w834) -> (1:w837:i32)  [unwired: 1 out]
                      n198 = Build Array(0.0, w822) -> (w821:dbl[])
                      n199 = Equal?(x=w837, y=w836) -> (x = y?=w827:bool)
                      n200 = Subtract(x=w835, y=w821) -> (x-y=w833:dbl[])
                      n201 = Insert Into Array(array=w834, new element=w833) -> (w832:dbl[][])  [unwired: 2 in]
                      n202 = case shown="True" w827 {
                        tunnel: [EstimateState."Calculando" ("Current State 2") EstimateState."Meio do campo" ("Current State 2")] -> w829
                        tunnel: [EstimateState."Meio superior" ("Current State 2") EstimateState."Aguardando próximo passo" ("Current State 2")] -> w828
                        frame False {
                        }
                        frame True {
                        }
                      }
                    }
                    frame "Meio do campo" {
                      w842 = 0.0
                      # "Erro entre ponto medido e o real"
                      # "Ponto real"
                      n203 = Matrix Size(0:w852) -> (1:w855:i32)  [unwired: 1 out]
                      n204 = Build Array(w842, w842) -> (w845:dbl[])
                      n205 = Equal?(x=w855, y=w854) -> (x = y?=w844:bool)
                      n206 = Subtract(x=w853, y=w845) -> (x-y=w851:dbl[])
                      n207 = Insert Into Array(array=w852, new element=w851) -> (w850:dbl[][])  [unwired: 2 in]
                      n208 = case shown="True" w844 {
                        tunnel: [EstimateState."Calculando" ("Current State 2") EstimateState."Centro do gol esquerdo" ("Current State 2")] -> w847
                        tunnel: [EstimateState."Meio do campo" ("Current State 2") EstimateState."Aguardando próximo passo" ("Current State 2")] -> w846
                        frame False {
                        }
                        frame True {
                        }
                      }
                    }
                    frame "Centro do gol esquerdo" {
                      n209 = Matrix Size(0:w869) -> (1:w872:i32)  [unwired: 1 out]
                      n210 = Equal?(x=w872, y=w871) -> (x = y?=w861:bool)
                      n211 = case shown="False" w861 {
                        tunnel: w870 -> [w884 _]
                        tunnel: w869 -> [w883 w886]
                        tunnel: [w876 w887] -> w865
                        tunnel: w868 -> [_ _]
                        tunnel: w867 -> [w880 _]
                        tunnel: [w876 w888] -> w866
                        tunnel: [w877 w886] -> w864
                        tunnel: [EstimateState."Calculando" ("Current State 2") w885] -> w863
                        tunnel: [EstimateState."Centro do gol esquerdo" ("Current State 2") w885] -> w862
                        frame False {
                          w876 = T4 [] ("covariance matrix V")
                          # "Ponto real"
                          # "Erro entre ponto medido e o real"
                          # "Don't have all points yet"
                          n212 = Divide(x=w880, y=-2.0) -> (x/y=w878:dbl)
                          n213 = Build Array(w878, 0.0 ("y")) -> (w881:dbl[])
                          n214 = Subtract(x=w884, y=w881) -> (x-y=w882:dbl[])
                          n215 = Insert Into Array(array=w883, new element=w882) -> (w877:dbl[][])  [unwired: 2 in]
                        }
                        frame True {
                          w885 = EstimateState."Terminado" ("Current State 2")
                          # "Estimate P"
                          # "Estimate R"
                          # "Last Point"
                          n216 = for {
                            tunnel: w886 -> [w895] mode=indexing
                            tunnel: [w890] -> w889 mode=indexing
                            w891 = 0.0
                            n217 = Index Array(array=w895) -> (element #1=w894:dbl, element #2=w893:dbl, element #3=w892:dbl)  [unwired: 3 in]
                            n218 = Build Array(w894, w891, w893, w891, w892, w891) -> (w890:dbl[])
                          }
                          n219 = call <vilib>:"Covariance Matrix.vi"("X"=w886) -> ("covariance matrix V"=w887:T4)  [unwired: 9 in, 1 out]
                          n220 = call <vilib>:"Covariance Matrix.vi"("X"=w889) -> ("covariance matrix V"=w888:T4)  [unwired: 9 in, 1 out]
                        }
                      }
                    }
                    frame "Terminado" {
                      w896 = TRUE
                      w897 = EstimateState."Terminado" ("Current State 2")
                    }
                  }
                }
              }
            }
          }
        }
      }
      n221 = feedback-in #5(w43) -> ()
    }
    frame Error {
    }
  }
  "error out" <- w24
  "Vision out" <- w22
  "Point Finished?" <- w3
  "Current State" <- w8
  "Camera Finished?" <- w2
  "covariance matrix P" <- w14
  "covariance matrix R" <- w16
  "Next State" <- w7
  n222 = feedback-in #1(w16) -> ()
  n223 = feedback-in #2(w14) -> ()
  n224 = feedback-in #3(w7) -> ()
  n225 = feedback-in #4(w8) -> ()
